vi "DBClose-Files.vi"(8 "error in (no error)":errorcluster, 11 "ProcessState in":T1) -> (0 "error out":errorcluster)   [LabVIEW 2015, in "FileHandler.lvlib"]
uses:
  FileHandler.lvlib
  controls/ProcessState.ctl
  <vilib>/drjdpowell/SQLite Library/SQL Connection/Connection.lvclass
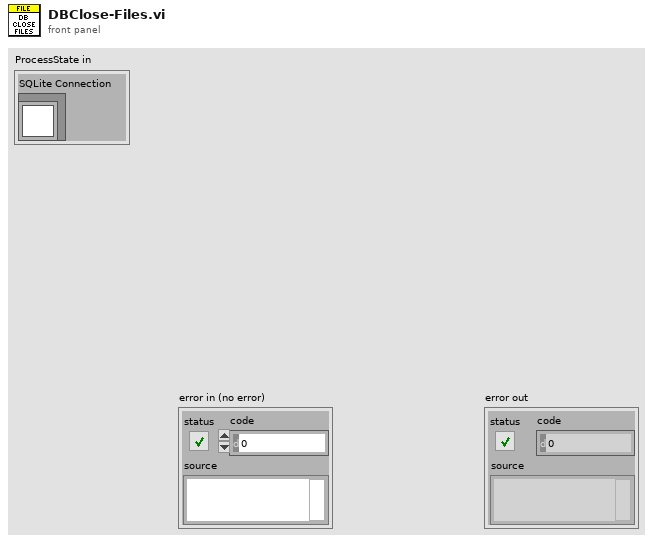
[diagram p1: front panel]
types:
  T1 = typedef "FileHandler.lvlib/ProcessState.ctl" = cluster{"SQLite Connection":refnum<class "Connection.lvclass">}
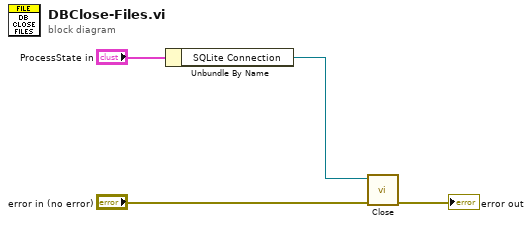
[diagram p0: block diagram]
diagram:
  n1 = Unbundle By Name("ProcessState in") -> ("SQLite Connection"=w2:refnum<class "Connection.lvclass">)
  n2 = call-dynamic "Close.vi"("error in (no error)"="error in (no error)", "SQLite Connection in"=w2) -> ("error out"=→"error out":errorcluster)  [unwired: 9 in]
